vi "testReadBlk.vi"() -> ()   [LabVIEW 2011]
panel:
  in  "SkipFrame":i32=8
  out "Image":T1(plugin-control)
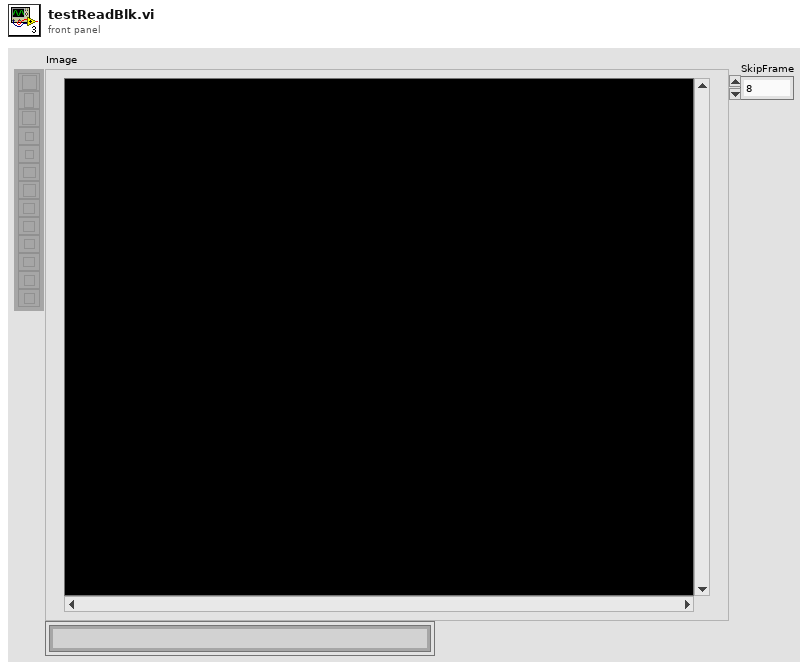
[diagram p1: front panel]
types:
  T1 = typedef "IMAQ Image.ctl" = refnum<image>
  T2 = typedef "Image Type" = u32
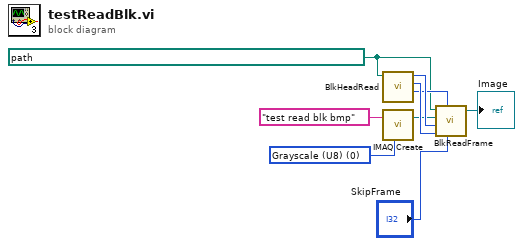
[diagram p0: block diagram]
diagram:
  w3 = T2 0 items=["Grayscale (U8)", "Grayscale (I16)", "Grayscale (SGL)", "Complex (CSG)", "RGB (U32)", "HSL (U32)", "RGB (U64)", "Grayscale (U16)"] ("Image Type")
  w6 = path "C:/Documents and Settings/pan/桌面/热成像/WriteTest4D.blk" ("BlkFilePath")
  n1 = call "BlkHeadRead.vi"("BlkFilePath"=w6) -> ("datatype"=w7:i32, "FrameHeight"=w8:i32, "FrameWidth"=w9:i32)  [unwired: 6 in, 2 out]
  n2 = call "IMAQ Create"("Image Name"="test read blk bmp", "Image Type"=w3) -> ("New Image"=w4:T1)  [unwired: 3 in, 1 out]
  n3 = call "BlkReadFrame.vi"("BlkFilePath"=w6, "datatype"=w7, "DST"=w4, "FrameWidth"=w9, "SkipFrame"="SkipFrame", "FrameHeight"=w8) -> ("Image out"=→"Image":T1)  [unwired: 2 in]
